vi "loop_n.vi"(0 "SIClass in":refnum<class "SIClass.lvclass">, 2 "Loop ID":enum16{"10", "20", "30", "40"}(ring), 3 "Input":dbl, 5 "error in (no error)":errorcluster) -> (14 "SIClass out":refnum<class "SIClass.lvclass">, 16 "Output":dbl, 19 "error out":errorcluster)   [LabVIEW 2022 SP3, in "SIClass.lvclass"]
uses:
  SIClass.lvclass
  SIClass.lvclass/SIClass.ctl
panel:
  in  ".A-SIG.OutLimMin":dbl
  in  "A-SIG.OutLimMax":dbl=1500.0
  in  "A-SIG.LL":dbl=-47.0
  in  "A-SIG.UL":dbl=1500.0
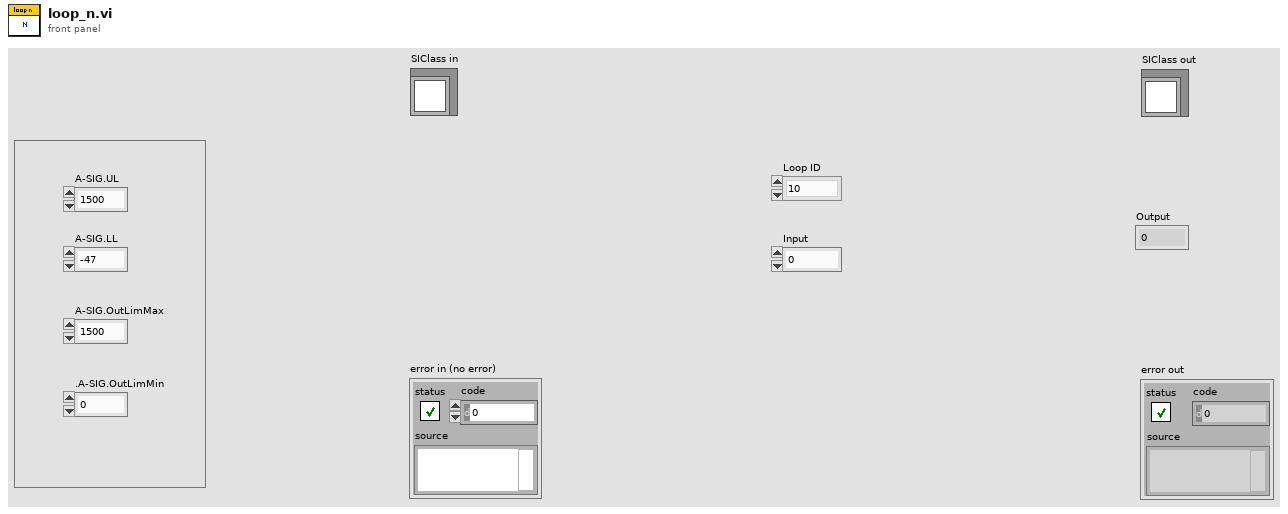
[diagram p1: front panel]
types:
  T1 = cluster{"A-SIG.UL":dbl, "A-SIG.LL":dbl, "A-SIG.OutLimMax":dbl, ".A-SIG.OutLimMin":dbl}
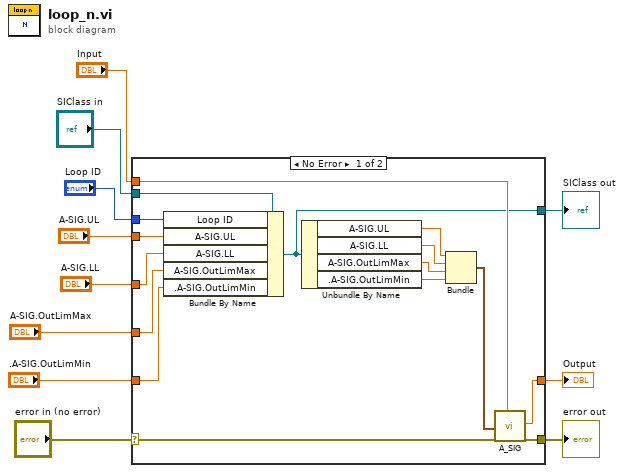
[diagram p0: block diagram]
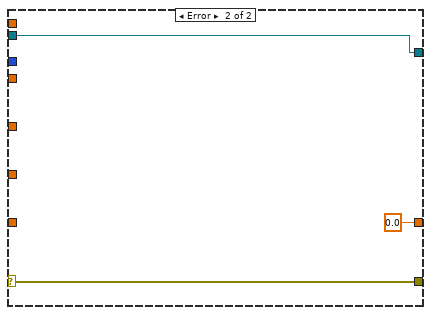
[diagram p2: hidden frame]
diagram:
  n1 = case shown="No Error" "error in (no error)" {
    selector: "error in (no error)" -> [w27 w30]
    tunnel: [w26 w30] -> w10
    tunnel: [w16 w29] -> w8
    tunnel: "SIClass in" -> [w19 w29]
    tunnel: "Input" -> [w24 _]
    tunnel: [w25 0.0 ("A_SIG_out")] -> w6
    tunnel: "Loop ID" -> [w18 _]
    tunnel: "A-SIG.UL" -> [w15 _]
    tunnel: "A-SIG.LL" -> [w14 _]
    tunnel: "A-SIG.OutLimMax" -> [w13 _]
    tunnel: ".A-SIG.OutLimMin" -> [w12 _]
    frame No Error {
      n2 = Bundle By Name(cluster=w19, "Loop ID"=w18, "A-SIG.UL"=w15, "A-SIG.LL"=w14, "A-SIG.OutLimMax"=w13, ".A-SIG.OutLimMin"=w12) -> (w16:refnum<class "SIClass.lvclass">)
      n3 = Unbundle By Name(w16) -> ("A-SIG.UL"=w23:dbl, "A-SIG.LL"=w22:dbl, "A-SIG.OutLimMax"=w21:dbl, ".A-SIG.OutLimMin"=w20:dbl)
      n4 = Bundle("A-SIG.UL"=w23, "A-SIG.LL"=w22, "A-SIG.OutLimMax"=w21, ".A-SIG.OutLimMin"=w20) -> (w17:T1)  [unwired: 1 in]
      n5 = call "A_SIG.vi"("Cluster"=w17, "error in (no error)"=w27, "Input"=w24) -> ("A_SIG_out"=w25:dbl, "error out"=w26:errorcluster)  [unwired: 15 in]
    }
    frame Error {
    }
  }
  "error out" <- w10
  "SIClass out" <- w8
  "Output" <- w6
